vi "Beginners Examples.vi"() -> ()   [LabVIEW 2017]
panel:
  in  "Input":dbl(slide) scale=-250.0..250.0
  out "What is this thing doing?":string
  in  "Switch Conversion":bool
  in  "stop":bool
  out "Result":dbl(slide) scale=0.0..212.0
  out "What do you want":string
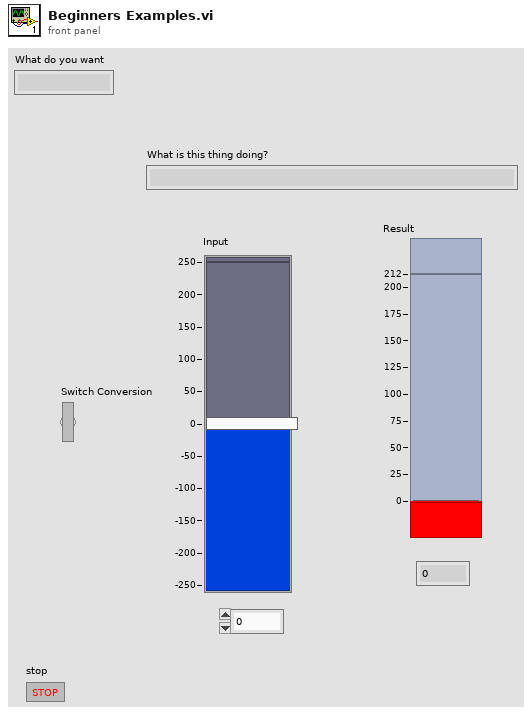
[diagram p1: front panel]
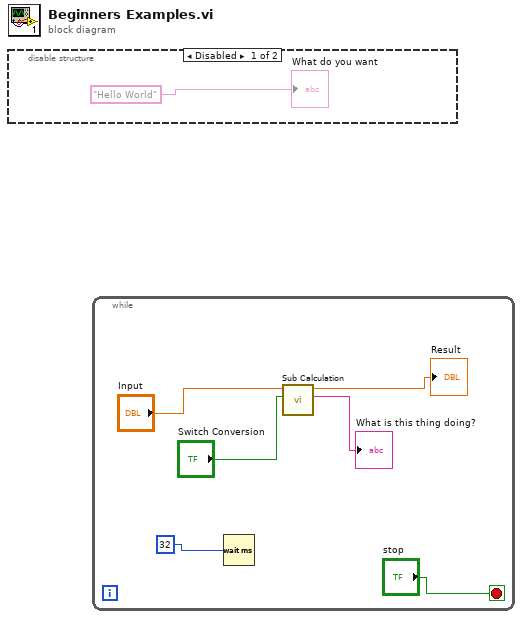
[diagram p0: block diagram]
diagram:
  n1 = disable-structure shown="Disabled" {
    frame Disabled {
      "What do you want" <- "Hello World"
    }
    frame Enabled {
    }
  }
  n2 = while {
    stop <- "stop" stop-if-true
    n3 = Wait (ms)(milliseconds to wait=32) -> ()  [unwired: 1 out]
    n4 = call "Sub Calculation.vi"("On/Off"="Switch Conversion", "Numeric in"="Input") -> ("String"=→"What is this thing doing?":string, "Numeric out"=→"Result":dbl)  [unwired: 8 in]
  }
